vi "Library Resolve Toolkit Directory.vi"(1 "VI name":string) -> (0 "toolkit directory":string)   [LabVIEW 2012]
doc: "Takes a VI name and returns the VI toolkit/library/class directory in lower case. This is done by extracting the substring before the first space and after any underscore that precedes the first space. This should work for VIs adhering to the VI class naming convention <prefix>_<toolkit>\\s<remainder of VI name> that is designed to avoid VI naming conflicts. Since all VIs of a particular toolkit/library/class are placed inside a subdirectory of the source tree with ditto name, this yields a directory name that can be used for path resolution."
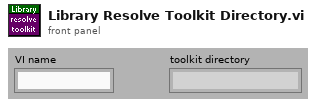
[diagram p1: front panel]
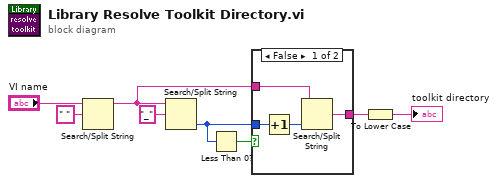
[diagram p0: block diagram]
diagram:
  n1 = Search/Split String(string="VI name", search string/char (-)=" ") -> (substring before match=w4:string)  [unwired: 1 in, 2 out]
  n2 = Search/Split String(string=w4, search string/char (-)="_") -> (offset of match=w3:i32)  [unwired: 1 in, 2 out]
  n3 = Less Than 0?(x=w3) -> (x < 0?=w5:bool)
  n4 = case shown="False" w5 {
    tunnel: w4 -> [w11 w13]
    tunnel: w3 -> [w12 _]
    tunnel: [w9 w13] -> w2
    frame False {
      n5 = Increment(x=w12) -> (x+1=w10:i32)
      n6 = Search/Split String(string=w11, offset (0)=w10) -> (match + rest of string=w9:string)  [unwired: 1 in, 2 out]
    }
    frame True {
    }
  }
  n7 = To Lower Case(string=w2) -> (all lower case string=→"toolkit directory":string)
